vi "Get Sender.vi"(11 "Msg in":refnum<class "Msg.lvclass">) -> (2 "Sender":refnum<class "Sender.lvclass">)   [LabVIEW 2021, in "jettl.lvlib" / "Msg.lvclass"]
uses:
  Msg.lvclass
  Sender/Sender/Sender.lvclass
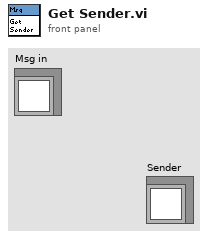
[diagram p1: front panel]
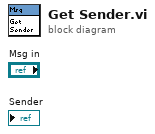
[diagram p0: block diagram]
diagram:
